vi "outlineWithMatlab.vi"() -> ()   [LabVIEW 2024]
panel:
  out "Array":path[][](array[path])
  out "String":string
  out "size(s)":i32
  out "appended path":path
  out "nume clase":string[](array[string])
  out "stripped path":path
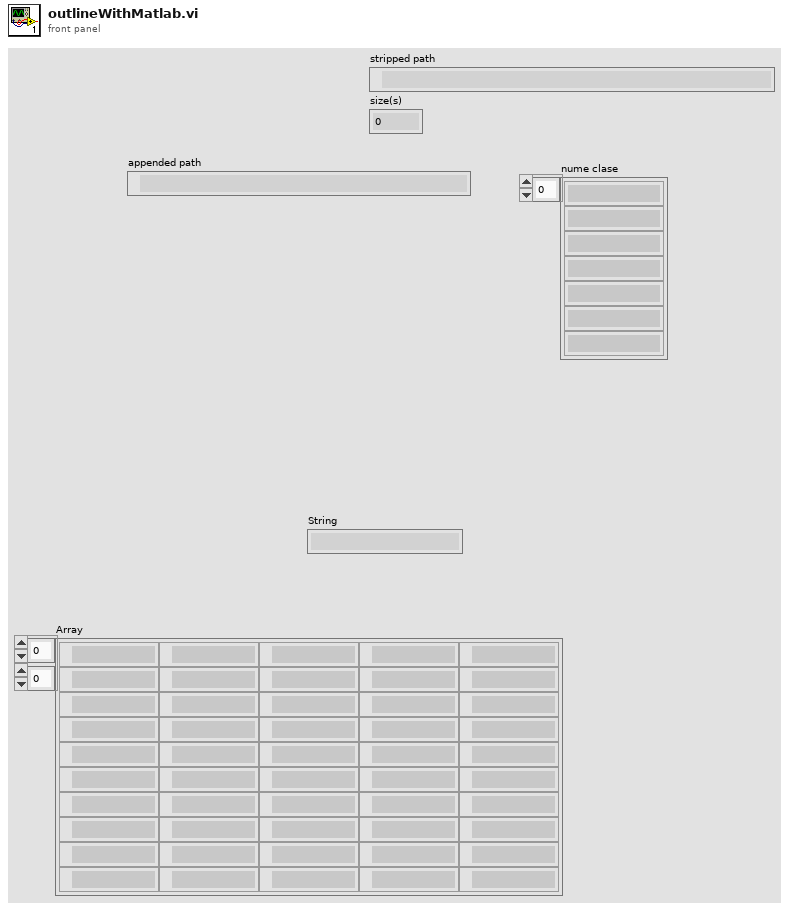
[diagram p1: front panel]
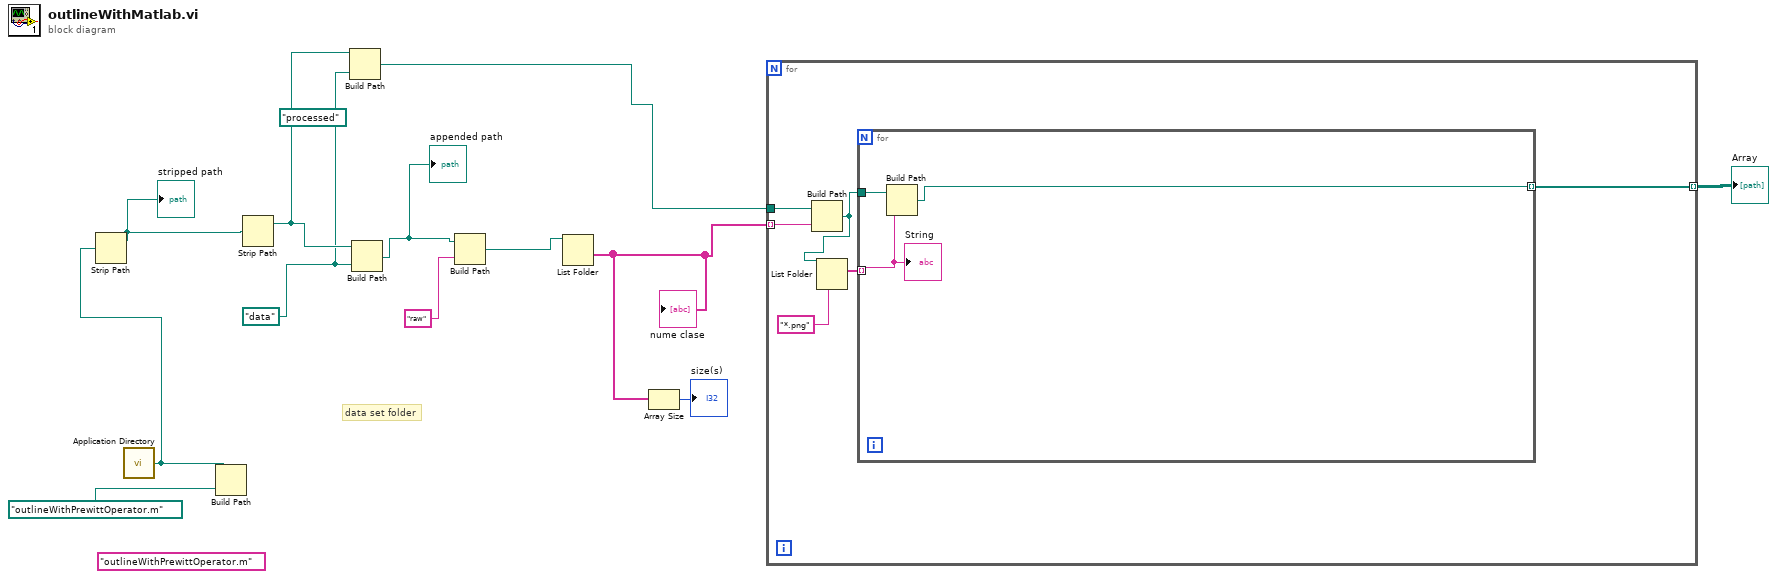
[diagram p0: block diagram]
diagram:
  (unwired) path "processed" ("name or relative path")
  w1 = path "data" ("name or relative path")
  (unwired) "outlineWithPrewittOperator.m"
  # "data set folder"
  n1 = call <vilib>:"Application Directory.vi"() -> ("Application Directory"=w11:path)
  n2 = Strip Path(path=w11) -> (stripped path=w10:path)  [unwired: 1 out]
  "stripped path" <- w10
  n3 = Build Path(base path=w11, name or relative path=path "outlineWithPrewittOperator.m") -> ()  [unwired: 1 out]
  n4 = Strip Path(path=w10) -> (stripped path=w4:path)  [unwired: 1 out]
  n5 = Build Path(base path=w4, name or relative path=w1) -> (appended path=w2:path)
  n6 = Build Path(base path=w4, name or relative path=w1) -> (appended path=w9:path)
  "appended path" <- w9
  n7 = Build Path(base path=w9, name or relative path="raw") -> (appended path=w7:path)
  n8 = List Folder(path=w7) -> (folder names=w5:string[])  [unwired: 3 in, 3 out]
  "nume clase" <- w5
  n9 = Array Size(array=w5) -> (size(s)=→"size(s)":i32)
  n10 = for {
    tunnel: w5 -> [w18] mode=indexing
    tunnel: w2 -> [w17]
    tunnel: [w13] -> w3 mode=indexing
    n11 = Build Path(base path=w17, name or relative path=w18) -> (appended path=w14:path)
    n12 = List Folder(path=w14, pattern="*.png") -> (filenames=w15:string[])  [unwired: 2 in, 3 out]
    n13 = for {
      tunnel: w15 -> [w20] mode=indexing
      tunnel: w14 -> [w21]
      tunnel: [w19] -> w13 mode=indexing
      n14 = Build Path(base path=w21, name or relative path=w20) -> (appended path=w19:path)
      "String" <- w20
    }
  }
  "Array" <- w3
